vi "Display time in seconds.vi"(11 "Event Date/Time":string="12-Mar-2018 11:55:33") -> (3 "Time in Seconds":i32)   [LabVIEW 2019]
doc: "Display Time in Seconds"
panel:
  out "Seconds":i32
  out "Minutes":i32
  out "Hours":i32
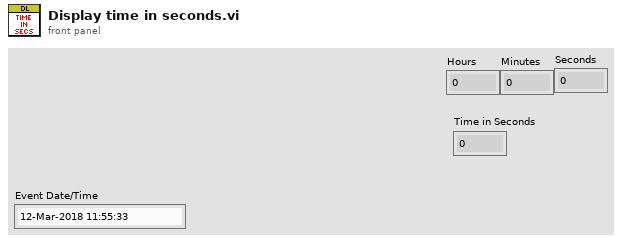
[diagram p1: front panel]
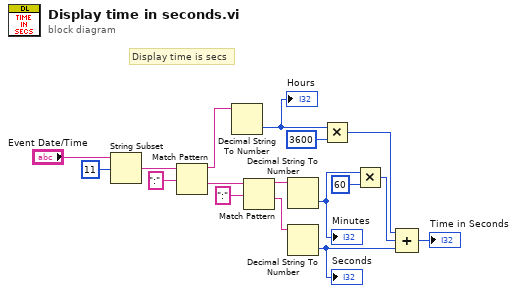
[diagram p0: block diagram]
diagram:
  # "Display time is secs"
  n1 = String Subset(string="Event Date/Time", offset (0)=11) -> (substring=w16:string)  [unwired: 1 in]
  n2 = Match Pattern(string=w16, regular expression=":") -> (before substring=w12:string, after substring=w13:string)  [unwired: 1 in, 2 out]
  n3 = Decimal String To Number(string=w12) -> (number=w6:i32)  [unwired: 2 in, 1 out]
  "Hours" <- w6
  n4 = Match Pattern(string=w13, regular expression=":") -> (before substring=w11:string, after substring=w10:string)  [unwired: 1 in, 2 out]
  n5 = Decimal String To Number(string=w11) -> (number=w9:i32)  [unwired: 2 in, 1 out]
  "Minutes" <- w9
  n6 = Decimal String To Number(string=w10) -> (number=w3:i32)  [unwired: 2 in, 1 out]
  "Seconds" <- w3
  n7 = Multiply(x=w6, y=3600) -> (x*y=w5:i32)
  n8 = Multiply(x=w9, y=60) -> (x*y=w4:i32)
  n9 = Compound Arithmetic op=ADD(w5, w4, w3) -> (→"Time in Seconds":i32)
